vi "Configure Frequency Limits.vi"(0 "VISA resource name":refnum<visa-resource-name>, 5 "Frequency Low Limit (40 Hz)":dbl=45.0 min=0.0 max=500.0 format="%.1f", 7 "Frequency High Limit (500 Hz)":dbl=500.0 min=0.0 max=500.0 format="%.1f", 11 "error in (no error)":errorcluster) -> (4 "VISA resource name out":refnum<visa-resource-name>, 15 "error out":errorcluster)   [LabVIEW 2020, in "eec 6700.lvlib"]
doc: "Configures the <B>Frequency Limits</B> of the power source instrument used for testing.\n\n<B>Range</B> : 45.0~500.0 Hz"
uses:
  <instrlib>/EEC6700LV-driver/eec 6700.lvlib
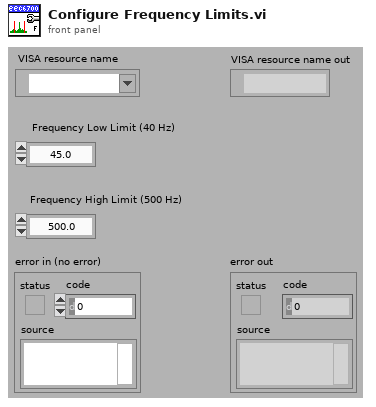
[diagram p1: front panel]
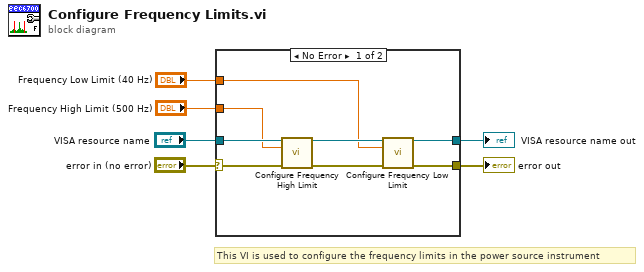
[diagram p0: block diagram]
diagram:
  # "This VI is used to configure the frequency limits in the power source instrument"
  n1 = case shown="No Error" "error in (no error)" {
    selector: "error in (no error)" -> [w9 w15]
    tunnel: "VISA resource name" -> [w14 w16]
    tunnel: [w13 w16] -> w5
    tunnel: [w12 w15] -> w4
    tunnel: "Frequency High Limit (500 Hz)" -> [w8 _]
    tunnel: "Frequency Low Limit (40 Hz)" -> [w7 _]
    frame No Error {
      n2 = call <instrlib>:"Configure Frequency High Limit.vi"("VISA resource name"=w14, "Frequency High Limit (500 Hz)"=w8, "error in (no error)"=w9) -> ("VISA resource name out"=w11:refnum<visa-resource-name>, "error out"=w10:errorcluster)  [unwired: 11 in]
      n3 = call <instrlib>:"Configure Frequency Low Limit.vi"("VISA resource name"=w11, "Frequency Low Limit (40 Hz)"=w7, "error in (no error)"=w10) -> ("VISA resource name out"=w13:refnum<visa-resource-name>, "error out"=w12:errorcluster)  [unwired: 11 in]
    }
    frame Error {
    }
  }
  "error out" <- w4
  "VISA resource name out" <- w5
